vi "resources_lua.vi"(5 "LuaVIEW reference":T1) -> (15 "error out":errorcluster)   [LabVIEW 2012]
doc: "Returns the resource base path of the server application as configured in the bootstrap script. By storing server-side resources inside the resources directory or its subdirectories the use of many different absolute paths can be avoided. Also, for security reasons, the remote file access GUIs limit themselves to accessing files inside the resource tree. The returned value reflects the value of a LabVIEW global so that the path can also be referenced from LabVIEW code.\nResults:\nstr:path"
uses:
  luaview/typedefs/t_LuaVIEW Reference.ctl
  library/glb_Library Configuration Globals.vi
  luaview/subvis/private/LuaVIEW Push (path).vi
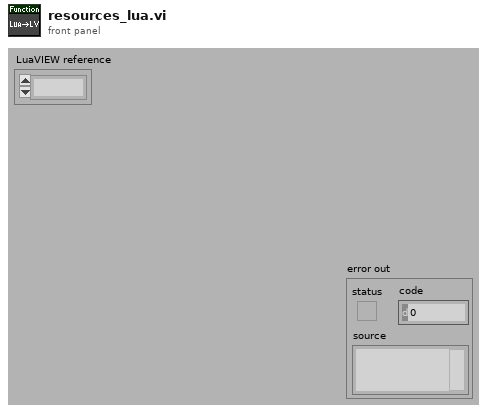
[diagram p1: front panel]
types:
  T1 = typedef "t_LuaVIEW Reference.ctl" = refnum<k1>
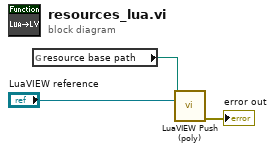
[diagram p0: block diagram]
diagram:
  n1 = global read "glb_Library Configuration Globals.vi" "resource base path"() -> (w2:path)
  n2 = call-poly "LuaVIEW Push (poly).vi"("path"=w2, "LuaVIEW reference in"="LuaVIEW reference") -> ("error out"=→"error out":errorcluster)  [unwired: 12 in, 1 out]
